vi "_JSON.Test.vi"() -> ()   [LabVIEW 2018]
panel:
  out "error out":errorcluster
  out "Data":dbl[](array[numeric])
  in  "path":string[](array[string])
  in  "String":string
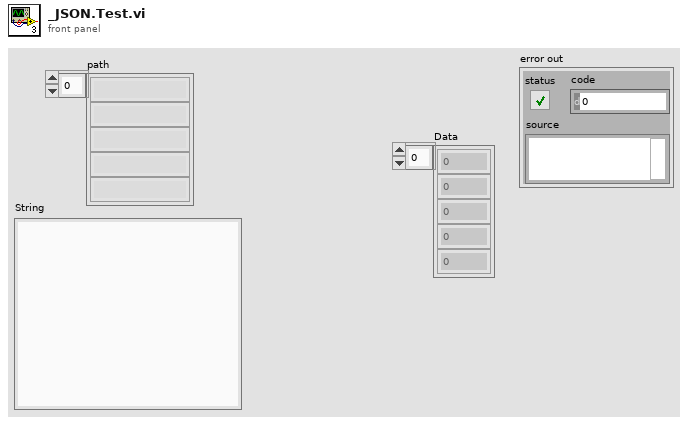
[diagram p1: front panel]
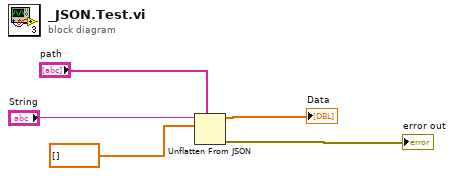
[diagram p0: block diagram]
diagram:
  n1 = Unflatten From JSON(path="path", JSON string="String", type and defaults=dbl[] [] ("Data")) -> (value=→"Data":dbl[], error out=→"error out":errorcluster)  [unwired: 4 in]
